vi "Draw Flat Bottom Filled Triangle.vi"(4 "Fill Colour":u32(colorbox), 8 "Point 3":T1, 9 "Point 2":T1, 10 "Point 1":T1, 11 "Pixel Data in":u32[][](array[numeric])) -> (3 "Pixel Data out":u32[][](array[numeric]))   [LabVIEW 2020, in "Raster.lvlib"]
uses:
  Raster.lvlib
  Point 2D.ctl
  <vilib>/Utility/High Resolution Relative Seconds.vi
  Utility/Utility.lvlib
panel:
  out "Delta Time [s]":dbl format="%.3p"
  out "x+y":i32
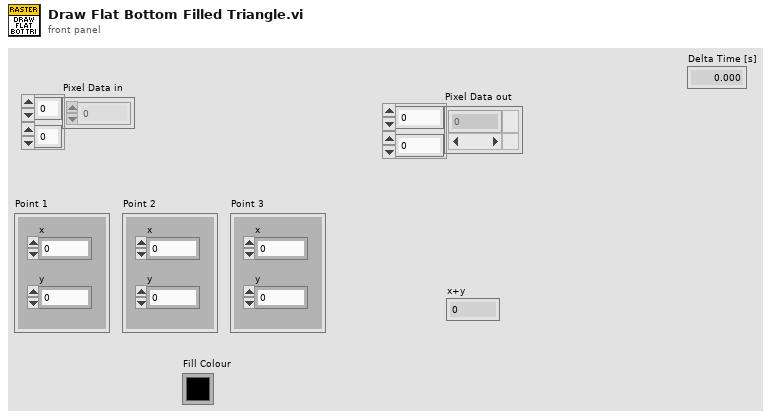
[diagram p1: front panel]
types:
  T1 = typedef "Raster.lvlib/Point 2D.ctl" = cluster{"x":i32, "y":i32}
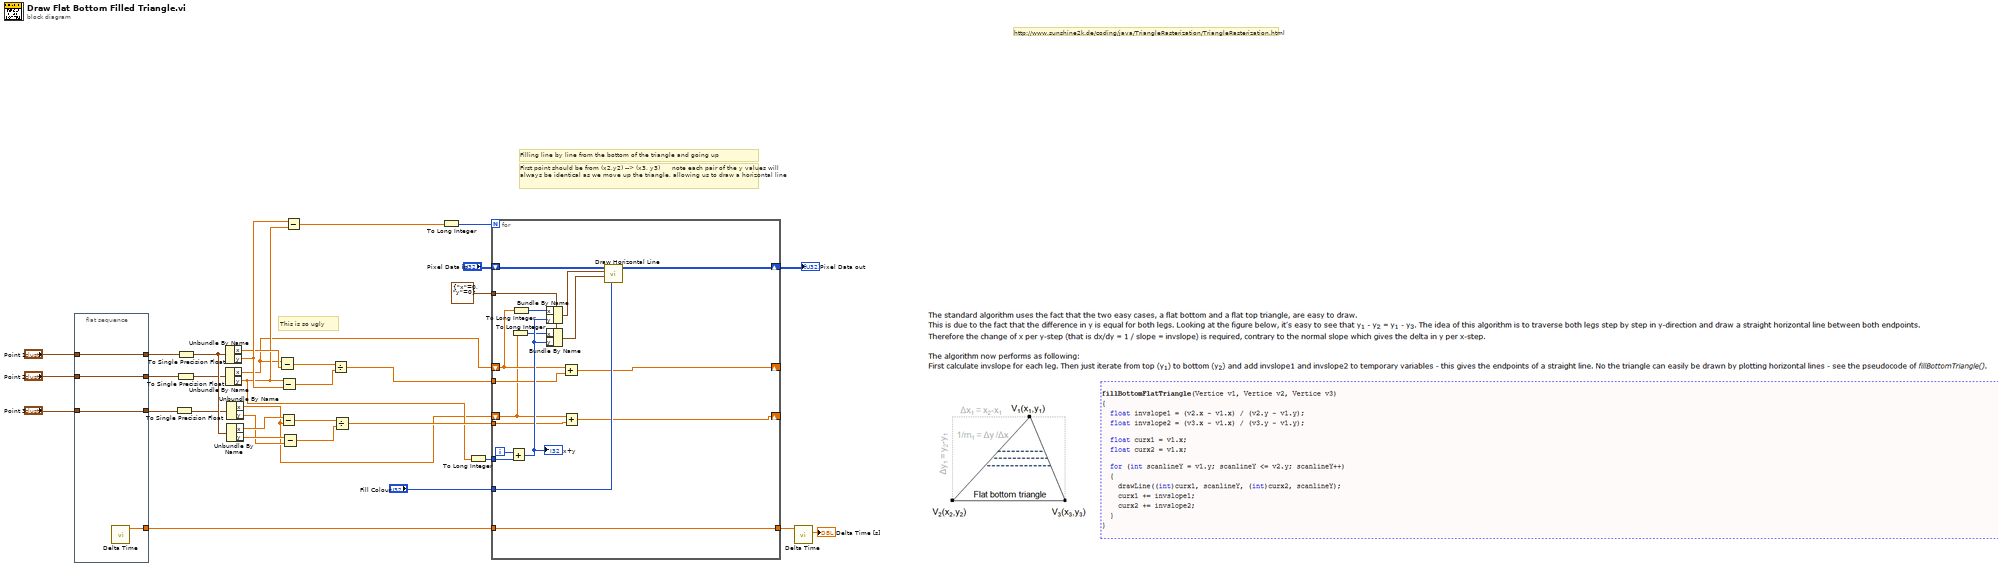
[diagram p0: block diagram]
diagram:
  # "This is so ugly"
  # "First point should be from (x2,y2) --> (x3, y3)      note each pair of the y values will always be identical as we move up the triangle, allowing us to draw a horizontal line"
  # "Filling line by line from the bottom of the triangle and going up"
  # "http://www.sunshine2k.de/coding/java/TriangleRasterization/TriangleRasterization.html"
  n1 = flat-sequence {
    tunnel: "Point 3" -> [w37]
    tunnel: [w37] -> w8
    tunnel: [w36] -> w7
    tunnel: "Point 2" -> [w36]
    tunnel: [w35] -> w5
    tunnel: "Point 1" -> [w35]
    tunnel: [w34] -> w3
    frame #0 {
      n2 = call "Delta Time.vi"() -> ("Relative Seconds Out"=w34:dbl)  [unwired: 10 in, 1 out]
    }
  }
  n3 = To Single Precision Float(number=w8) -> (single precision float=w26:cluster{"x":sgl, "y":sgl})
  n4 = To Single Precision Float(number=w7) -> (single precision float=w27:cluster{"x":sgl, "y":sgl})
  n5 = To Single Precision Float(number=w5) -> (single precision float=w28:cluster{"x":sgl, "y":sgl})
  n6 = Unbundle By Name(w28) -> ("x"=w17:sgl, "y"=w21:sgl)
  n7 = Unbundle By Name(w27) -> ("x"=w15:sgl, "y"=w16:sgl)
  n8 = Unbundle By Name(w26) -> ("x"=w13:sgl, "y"=w14:sgl)
  n9 = Unbundle By Name(w28) -> ("x"=w29:sgl, "y"=w31:sgl)
  n10 = Subtract(x=w15, y=w17) -> (x-y=w32:sgl)
  n11 = Subtract(x=w29, y=w13) -> (x-y=w30:sgl)
  n12 = Subtract(x=w16, y=w21) -> (x-y=w24:sgl)
  n13 = Subtract(x=w31, y=w14) -> (x-y=w25:sgl)
  n14 = Subtract(x=w21, y=w16) -> (x-y=w12:sgl)
  n15 = Divide(x=w32, y=w24) -> (x/y=w19:sgl)
  n16 = Divide(x=w30, y=w25) -> (x/y=w18:sgl)
  n17 = To Long Integer(number=w12) -> (32bit integer=w11:i32)
  n18 = To Long Integer(number=w16) -> (32bit integer=w20:i32)
  n19 = for {
    N: w11 -> [_]
    shift-right: [w39] -> w10
    shift-left: "Pixel Data in" -> [w55]
    tunnel: T1 {"x"=0, "y"=0} ("Point 1") -> [w54]
    tunnel: "Fill Colour" -> [w51]
    shift-right: [w42] -> _
    shift-left: w15 -> [w45]
    shift-right: [w43] -> _
    shift-left: w13 -> [w40]
    tunnel: w20 -> [w47]
    tunnel: w19 -> [w44]
    tunnel: w18 -> [w41]
    tunnel: [w38] -> w2
    tunnel: w3 -> [w38]
    i -> [w49]
    n20 = Add(x=w49, y=w47) -> (x+y=w48:i32)
    "x+y" <- w48
    n21 = To Long Integer(number=w40) -> (32bit integer=w46:i32)
    n22 = To Long Integer(number=w45) -> (32bit integer=w50:i32)
    n23 = Bundle By Name(cluster=w54, "x"=w50, "y"=w48) -> (w53:T1)
    n24 = Bundle By Name(cluster=w54, "x"=w46, "y"=w48) -> (w52:T1)
    n25 = Add(x=w45, y=w44) -> (x+y=w42:sgl)
    n26 = Add(x=w40, y=w41) -> (x+y=w43:sgl)
    n27 = call "Draw Horizontal Line.vi"("Colour"=w51, "Point 2"=w52, "Point 1"=w53, "Pixel Data in"=w55) -> ("Pixel Data out"=w39:u32[][])  [unwired: 7 in]
  }
  "Pixel Data out" <- w10
  n28 = call "Delta Time.vi"("Relative Seconds In"=w2) -> ("Delta Time [s]"=→"Delta Time [s]":dbl)  [unwired: 9 in, 1 out]
